vi "Read Latest Messages Data.vi"(8 "error in (no error)":errorcluster, 11 "Debugger In":refnum<class "Debugger.lvclass">) -> (0 "error out":errorcluster, 2 "Latest Messages":map{string, refnum<class "Debug Data.lvclass">}(c390), 3 "Debugger Out":refnum<class "Debugger.lvclass">)   [LabVIEW 2020, in "Debugger.lvclass"]
uses:
  Debugger.lvclass
  Debug Data/Debug Data.lvclass
  Debug Latest Message/Debug Latest Message.lvclass
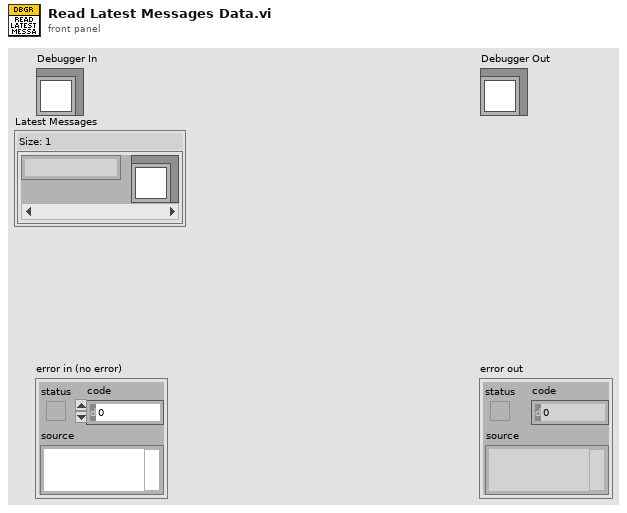
[diagram p1: front panel]
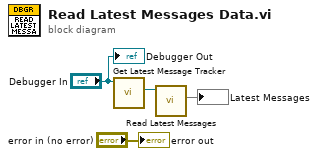
[diagram p0: block diagram]
diagram:
  n1 = call "Get Latest Message Tracker.vi"("Debugger in"="Debugger In") -> ("Latest Message Tracker"=w1:refnum<class "Debug Latest Message.lvclass">)  [unwired: 8 in, 2 out]
  n2 = call "Read Latest Messages.vi"("Debug Latest Message in"=w1) -> ("Latest Messages"=→"Latest Messages":map{string, refnum<class "Debug Data.lvclass">})  [unwired: 8 in, 2 out]
  "error out" <- "error in (no error)"
  "Debugger Out" <- "Debugger In"
